vi "UDPSender.vi"(9 "port":u16, 10 "RoboRIO IP":string, 11 "UDP Network Connection in":refnum<k16>) -> (3 "UDP Network Connection out":refnum<k16>)   [LabVIEW 2015]
uses:
  GlobalVars.vi
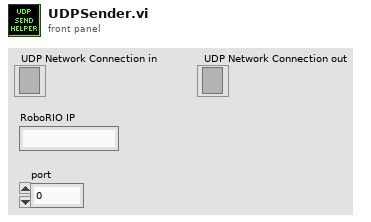
[diagram p1: front panel]
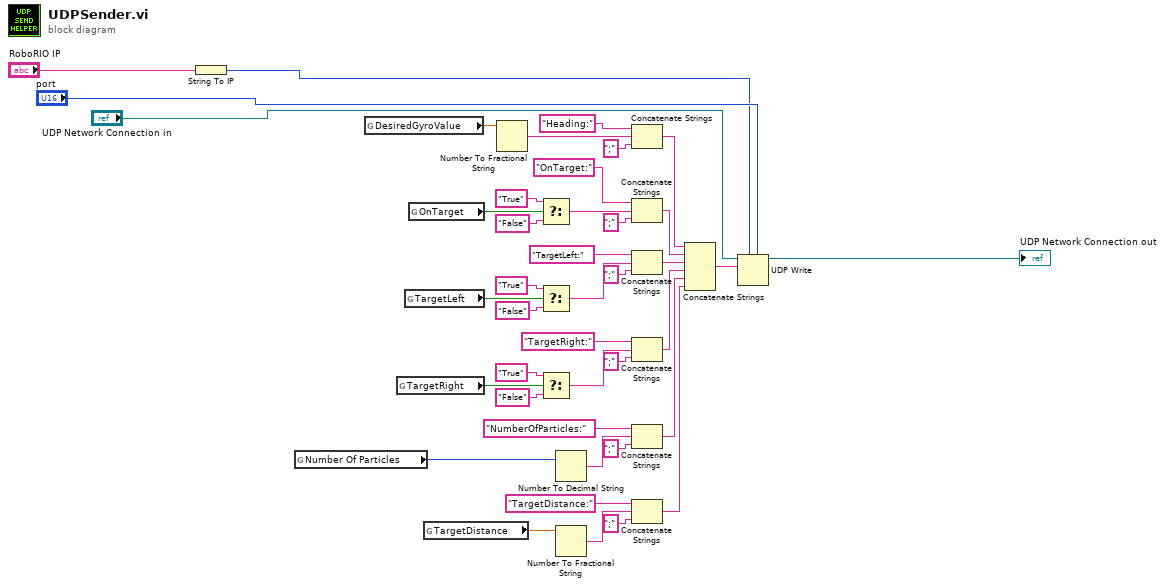
[diagram p0: block diagram]
diagram:
  n1 = String To IP(1:"RoboRIO IP") -> (0:w3:u32)
  n2 = global read "GlobalVars.vi" "Number Of Particles"() -> (w42:i32)
  n3 = global read "GlobalVars.vi" "DesiredGyroValue"() -> (w6:dbl)
  n4 = global read "GlobalVars.vi" "TargetRight"() -> (w20:bool)
  n5 = global read "GlobalVars.vi" "TargetLeft"() -> (w15:bool)
  n6 = global read "GlobalVars.vi" "OnTarget"() -> (w10:bool)
  n7 = global read "GlobalVars.vi" "TargetDistance"() -> (w41:dbl)
  n8 = Number To Fractional String(number=w6) -> (F-format string=w7:string)  [unwired: 3 in]
  n9 = Select(t="True" ("string"), s=w10, f="False") -> (s? t:f=w11:string)
  n10 = Select(t="True" ("string"), s=w15, f="False") -> (s? t:f=w16:string)
  n11 = Select(t="True" ("string"), s=w20, f="False") -> (s? t:f=w21:string)
  n12 = Number To Decimal String(number=w42) -> (decimal integer string=w35:string)  [unwired: 1 in]
  n13 = Number To Fractional String(number=w41) -> (F-format string=w40:string)  [unwired: 3 in]
  n14 = Concatenate Strings("Heading:" ("string"), w7, ";" ("string")) -> (w28:string)
  n15 = Concatenate Strings("OnTarget:" ("string"), w11, ";" ("string")) -> (w29:string)
  n16 = Concatenate Strings("TargetLeft:" ("string"), w16, ";" ("string")) -> (w30:string)
  n17 = Concatenate Strings("TargetRight:" ("string"), w21, ";" ("string")) -> (w31:string)
  n18 = Concatenate Strings("NumberOfParticles:" ("string"), w35, ";" ("string")) -> (w36:string)
  n19 = Concatenate Strings("TargetDistance:" ("string"), w40, ";" ("string")) -> (w39:string)
  n20 = Concatenate Strings(w28, w29, w30, w31, w36, w39) -> (w32:string)
  n21 = UDP Write(address=w3, port or service name="port", connection ID="UDP Network Connection in", data in=w32) -> (3:→"UDP Network Connection out":refnum<k16>)  [unwired: 2 in, 1 out]
